vi "Justification.vi"() -> ()   [LabVIEW 2013]
doc: "This VI demostrate how to justify a text string."
panel:
  out "Justification style":enum16{"Left", "Center", "Right"}(ring)
  in  "stop":bool
  out "String":string
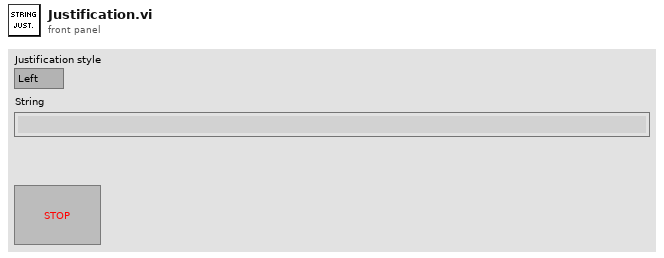
[diagram p1: front panel]
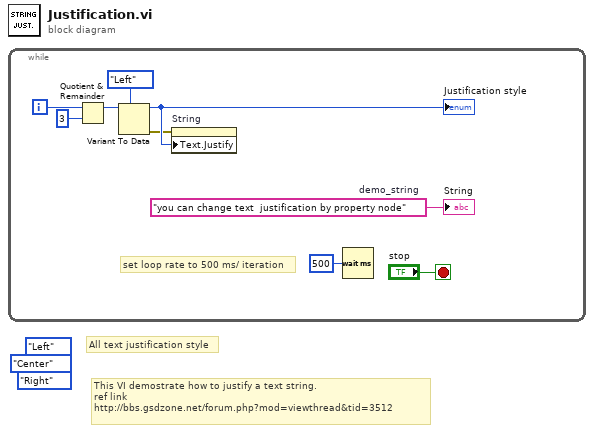
[diagram p0: block diagram]
diagram:
  (unwired) enum16{"Left", "Center", "Right"}."Right" ("Text.Justification")
  (unwired) enum16{"Left", "Center", "Right"}."Center" ("Text.Justification")
  (unwired) enum16{"Left", "Center", "Right"}."Left" ("Text.Justification")
  # "This VI demostrate how to justify a text string.\nref link\nhttp://bbs.gsdzone.net/forum.php?mod=viewthread&tid=3512"
  # "All text justification style"
  n1 = while {
    i -> [w9]
    stop <- "stop" stop-if-true
    w7 = "you can change text  justification by property node"  # demo_string
    # "set loop rate to 500 ms/ iteration"
    n2 = Quotient & Remainder(x=w9, y=3) -> (x-y*floor(x/y)=w4:i32)  [unwired: 1 out]
    n3 = Variant To Data(type=enum16{"Left", "Center", "Right"}."Left" ("Text.Justification"), Variant=w4) -> (data=w2:enum16{"Left", "Center", "Right"}, error out=w1:errorcluster)  [unwired: 1 in]
    "Justification style" <- w2
    n4 = property on="String" class="Str"(error in=w1, "Text.Justify"=w2) -> ()  [unwired: 1 in, 2 out]
    n5 = Wait (ms)(milliseconds to wait=u32 500) -> ()  [unwired: 1 out]
    "String" <- w7
  }
